vi "Untitled 2 (SubVI)RIJDEN.vi"(10 "digital in":bool[](array[boolean]), 11 "stop":bool) -> ()   [LabVIEW 2018]
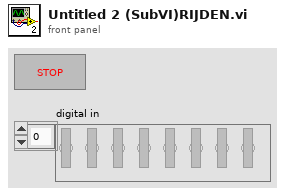
[diagram p1: front panel]
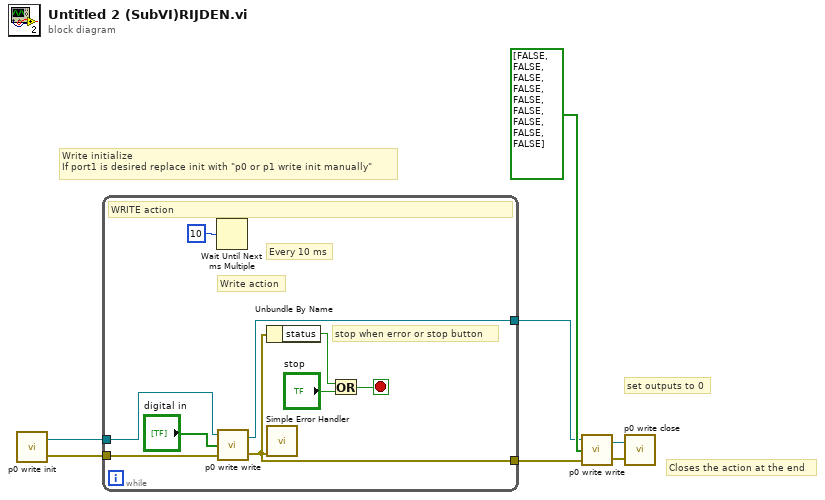
[diagram p0: block diagram]
diagram:
  # "set outputs to 0"
  # "Closes the action at the end"
  # "Write initialize\nIf port1 is desired replace init with \"p0 or p1 write init manually\""
  n1 = call "p0 write init.vi"() -> ("error out"=w6:errorcluster, "task out"=w5:refnum<k21>)
  n2 = while {
    tunnel: w5 -> [w16]
    tunnel: [w15] -> w1
    tunnel: w6 -> [w14]
    tunnel: [w9] -> w2
    stop <- w10 stop-if-true
    # "stop when error or stop button"
    # "Every 10 ms"
    # "Write action"
    # "WRITE action"
    n3 = Wait Until Next ms Multiple(millisecond multiple=u32 10) -> ()  [unwired: 1 out]
    n4 = call "p0 write write.vi"("error in"=w14, "digital out"="digital in", "task/channels in"=w16) -> ("error out"=w9:errorcluster, "task out"=w15:refnum<k21>)
    n5 = Unbundle By Name(w9) -> ("status"=w8:bool)
    n6 = call <vilib>:"Simple Error Handler.vi"("error in (no error)"=w9) -> ()  [unwired: 4 in, 5 out]
    n7 = Or(x=w8, y="stop") -> (x .or. y?=w10:bool)
  }
  n8 = call "p0 write write.vi"("error in"=w2, "digital out"=bool[] [FALSE, FALSE, FALSE, FALSE, FALSE, FALSE, FALSE, FALSE, FALSE], "task/channels in"=w1) -> ("error out"=w4:errorcluster, "task out"=w3:refnum<k21>)
  n9 = call "p0 write close.vi"("error in"=w4, "task/channels in"=w3) -> ()
